vi "APS relative linear move.vi"(7 "Max_Linear_Speed":i32, 8 "error in (no error)":errorcluster caption="错误输入（无错误）", 9 "Distance_Array":i32, 10 "Axis_ID_Array":i32, 11 "Dimension":i32) -> (0 "error out":errorcluster caption="错误输出", 1 "Distance_Array out":i32, 2 "Axis_ID_Array out":i32, 3 "function return":i32)   [LabVIEW 2011, in "APS168.lvlib"]
doc: "I32 FNTYPE APS_relative_linear_move( I32 Dimension, I32 *Axis_ID_Array, I32 *Distance_Array, I32 Max_Linear_Speed );"
uses:
  APS168.lvlib
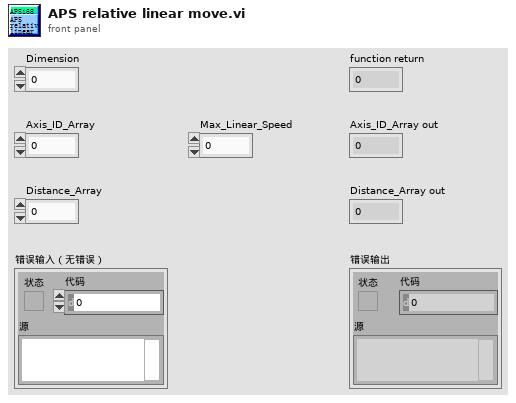
[diagram p1: front panel]
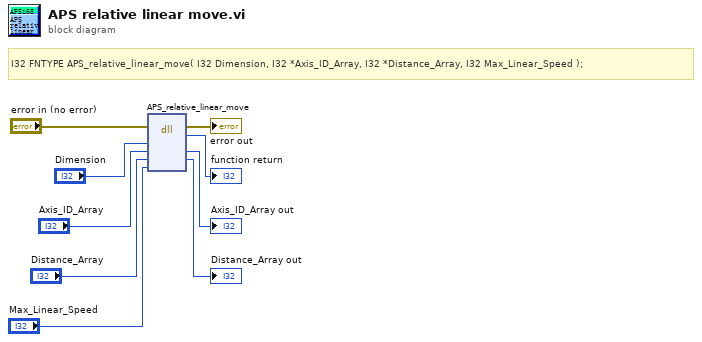
[diagram p0: block diagram]
diagram:
  # "I32 FNTYPE APS_relative_linear_move( I32 Dimension, I32 *Axis_ID_Array, I32 *Distance_Array, I32 Max_Linear_Speed );"
  n1 = dll-call lib="PTH1Labs E软件ADLINK 204CAPS_1_7_1_LIB line 连续运动204APS168.*" fn="APS_relative_linear_move"(error in="error in (no error)", "Dimension"="Dimension", "Axis_ID_Array"="Axis_ID_Array", "Distance_Array"="Distance_Array", "Max_Linear_Speed"="Max_Linear_Speed") -> (error out=→"error out":errorcluster, →"function return":i32, "Axis_ID_Array"=→"Axis_ID_Array out":i32, "Distance_Array"=→"Distance_Array out":i32)  [unwired: 4 in, 1 out]
